vi "01 - Offline client lifecycle.vi"() -> ()   [LabVIEW 2020]
uses:
  client/client.lvlib
panel:
  out "base url":string
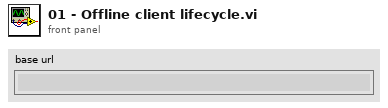
[diagram p1: front panel]
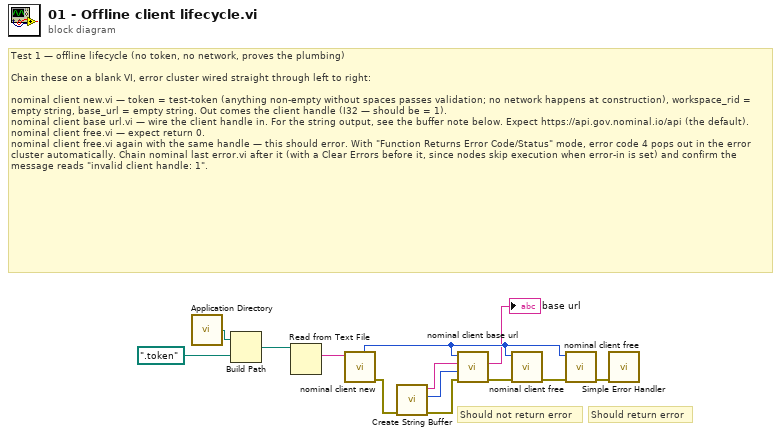
[diagram p0: block diagram]
diagram:
  # "Should not return error"
  # "Should return error"
  # "Test 1 — offline lifecycle (no token, no network, proves the plumbing)\n\nChain these on a blank VI, error cluster wired straight through left to right:\n\nnominal client new.vi — token = test-token (anything non-empty without spaces passes validation; no network happens at construction), workspace_rid = empty string, base_url = empty string. Out comes the client handle (I32 — should be = 1).\nnominal client base url.vi — wire the client handle in. For the string output, see the buffer note below. Expect https://api.gov.nominal.io/api (the default).\nnominal client free.vi — expect return 0.\nnominal client free.vi again with the same handle — this should error. With \"Function Returns Error Code/Status\" mode, error code 4 pops out in the error cluster automatically. Chain nominal last error.vi after it (with a Clear Errors before it, since nodes skip execution when error-in is set) and confirm the message reads \"invalid client handle: 1\"."
  n1 = call <vilib>:"Application Directory.vi"() -> ("Application Directory"=w8:path)
  n2 = Build Path(base path=w8, name or relative path=path ".token") -> (appended path=w6:path)
  n3 = Read from Text File(file (use dialog)=w6) -> (text=w5:string)  [unwired: 3 in, 3 out]
  n4 = call "nominal client new.vi"("token"=w5) -> ("error out"=w2:errorcluster, "out_client out"=w13:i32)  [unwired: 8 in, 1 out]
  n5 = call "Create String Buffer.vi"("error in"=w2) -> ("error out"=w1:errorcluster, "dub Buffer Size"=w3:i32, "String Buffer"=w4:string)  [unwired: 8 in]
  n6 = call "nominal client base url.vi"("error in (no error)"=w1, "cap"=w3, "buf"=w4, "client"=w13) -> ("error out"=w12:errorcluster, "buf out"=→"base url":string)  [unwired: 4 in, 2 out]
  n7 = call "nominal client free.vi"("error in (no error)"=w12, "client"=w13) -> ("error out"=w11:errorcluster)  [unwired: 8 in, 1 out]
  n8 = call "nominal client free.vi"("error in (no error)"=w11, "client"=w13) -> ("error out"=w9:errorcluster)  [unwired: 8 in, 1 out]
  n9 = call <vilib>:"Simple Error Handler.vi"("error in (no error)"=w9) -> ()  [unwired: 4 in, 5 out]
